vi "Device Identification.vi"(8 "error in":errorcluster, 11 "VISA resource name":refnum<visa-resource-name>) -> (0 "error out":errorcluster, 2 "Device Identification":string, 3 "VISA resource name out":refnum<visa-resource-name>)   [LabVIEW 2011, in "DMM4.lvlib"]
uses:
  <instrlib>/DMM4/DMM4.lvlib
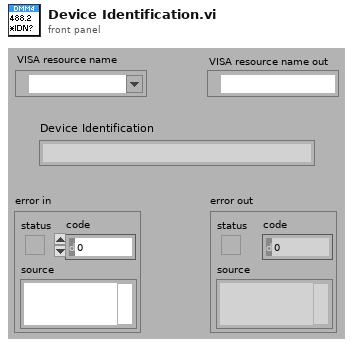
[diagram p1: front panel]
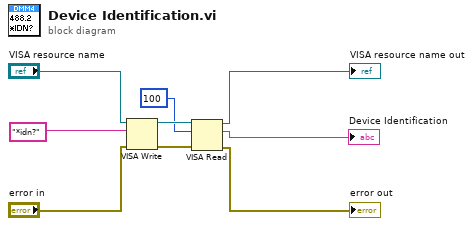
[diagram p0: block diagram]
diagram:
  n1 = VISA Write(VISA resource name="VISA resource name", write buffer="*idn?", error in (no error)="error in") -> (VISA resource name out=w7:refnum<visa-resource-name>, error out=w6:errorcluster)  [unwired: 1 out]
  n2 = VISA Read(VISA resource name=w7, byte count=u32 100, error in (no error)=w6) -> (VISA resource name out=→"VISA resource name out":refnum<visa-resource-name>, read buffer=→"Device Identification":string, error out=→"error out":errorcluster)  [unwired: 1 out]
